vi "test_5772_stage2.vi"() -> ()   [LabVIEW 2013]
uses:
  <vilib>/measure/maspectr.llb/Power Spectrum and PSD Export Mode.ctl
  <vilib>/measure/maspectr.llb/FFT Power Spectrum and PSD for 1 Chan (CDB).vi
  <vilib>/measure/NI_MAPro.lvlib
  <vilib>/rvi/FXPMathLib/FxpInterpret/XNode/nifxpmath_Interpret.xnode
panel:
  out "size before":i32
  out "data in":dbl[](graph)
  out "size after":i32
  out "power spectrum after":cluster{"f0":dbl, "df":dbl, "magnitude":dbl[]}(graph)
  out "power spectrum bef":cluster{"f0":dbl, "df":dbl, "magnitude":dbl[]}(graph)
  out "data out":i16[](graph)
  out "Iteration":i32
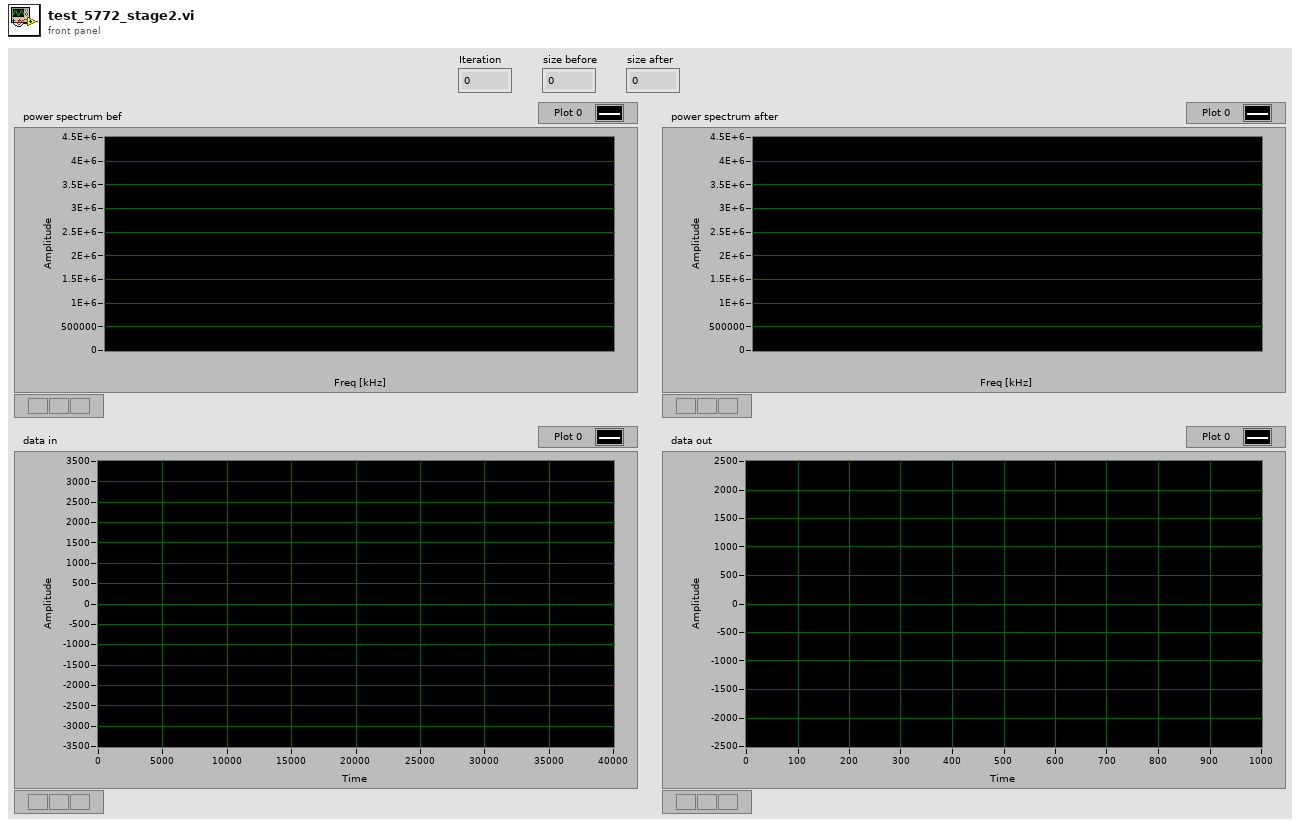
[diagram p1: front panel]
types:
  T1 = typedef "NI_MAPro.lvlib/Power Spectrum and PSD Export Mode.ctl" = u16
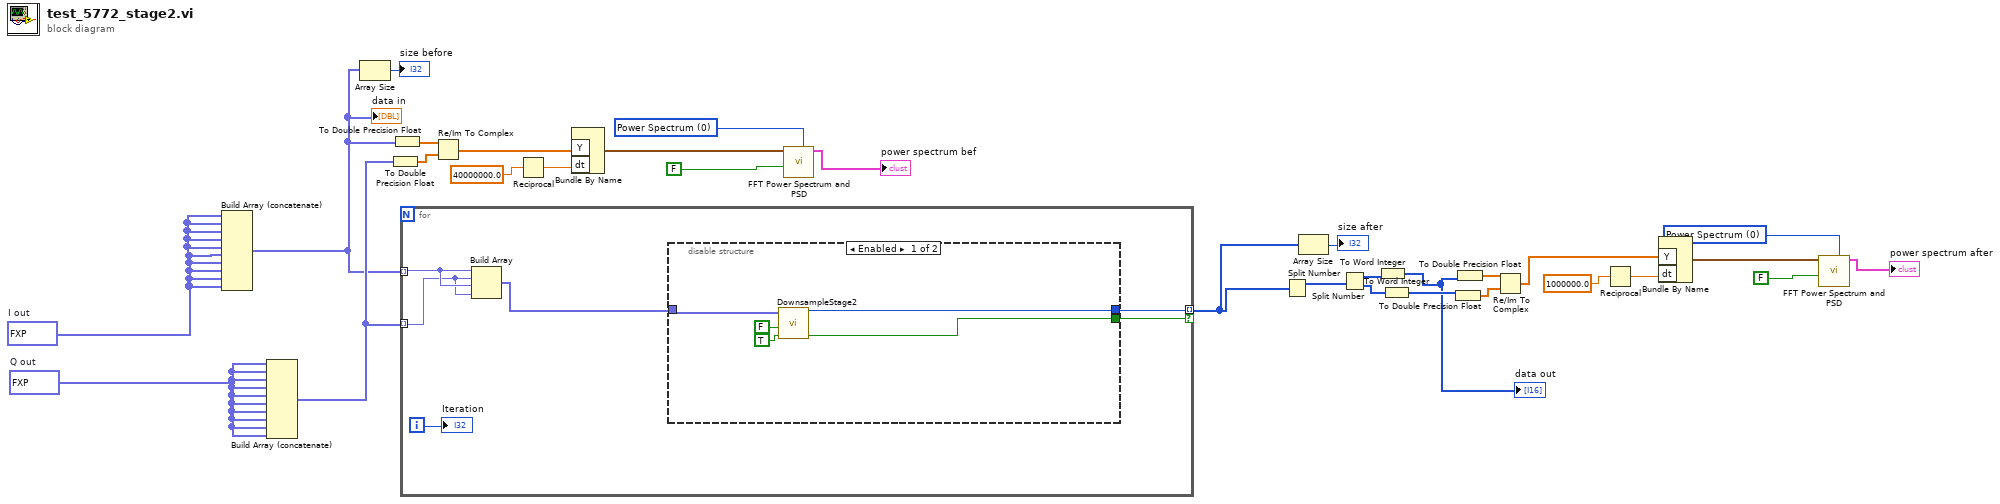
[diagram p0: block diagram]
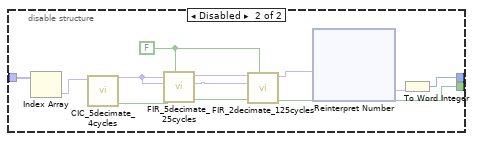
[diagram p2: hidden frame]
diagram:
  w4 = fxp[] data[31948B]  # Q out
  w5 = fxp[] data[31948B]  # I out
  w16 = T1 0 items=["Power Spectrum", "Power Spectral Density"] ("export mode")
  w30 = T1 0 items=["Power Spectrum", "Power Spectral Density"] ("export mode")
  n1 = Build Array (concatenate)(w5, w5, w5, w5, w5, w5, w5, w5, w5, w5) -> (w1:fxp<+/-,16,14>[])
  "data in" <- w1
  n2 = Build Array (concatenate)(w4, w4, w4, w4, w4, w4, w4, w4, w4, w4) -> (w6:fxp<+/-,16,14>[])
  n3 = Array Size(array=w1) -> (size(s)=→"size before":i32)
  n4 = To Double Precision Float(number=w6) -> (double precision float=w23:dbl[])
  n5 = To Double Precision Float(number=w1) -> (double precision float=w24:dbl[])
  n6 = for {
    tunnel: w1 -> [w36] mode=indexing
    tunnel: w6 -> [w35] mode=indexing
    tunnel: [w32] -> w3 mode=indexing if=w31
    i -> [w34]
    n7 = Build Array(w36, w35, w36, w35) -> (w33:fxp<+/-,16,14>[])
    n8 = disable-structure shown="Enabled" {
      disable-tunnel: w33 -> [w39 w48]
      disable-tunnel: [w40 w46] -> w31
      disable-tunnel: [w37 w43] -> w32
      frame Enabled {
        n9 = call "DownsampleStage2.vi"("valid in"=TRUE, "reset"=FALSE, "Element"=w39) -> ("valid out"=w40:bool, "Element"=w37:u64)  [unwired: 7 in]
      }
      frame Disabled {
        w50 = FALSE ("reset")
        n10 = Index Array(array=w48) -> (element=w47:fxp<+/-,16,14>)  [unwired: 1 in]
        n11 = call "CIC_5decimate_4cycles.vi"("Data in"=w47) -> ("valid out"=w53:bool, "Data out"=w54:fxp<+/-,16,14>, "valid in"=w42:bool)  [unwired: 7 in, 1 out]
        n12 = call "FIR_5decimate_25cycles.vi"("reset"=w50, "valid in"=w53, "Q in"=w54, "I in"=w54) -> ("valid out"=w49:bool, "Q out"=w51:fxp<+/-,16,14>, "I out"=w52:fxp<+/-,16,14>)  [unwired: 4 in, 1 out]
        n13 = call "FIR_2decimate_125cycles.vi"("reset"=w50, "valid in"=w49, "Q in"=w51, "I in"=w52) -> ("valid out"=w46:bool, "I out"=w44:fxp<+/-,16,14>)  [unwired: 4 in, 2 out]
        n14 = xnode "Reinterpret Number"("x"=w44) -> ("y"=w45:fxp<+/-,16,16>)
        n15 = To Word Integer(number=w45) -> (16bit integer=w43:i16)
      }
    }
    "Iteration" <- w34
  }
  n16 = Re/Im To Complex(1:w23, 2:w24) -> (0:w22:cdb[])
  n17 = Reciprocal(x=40000000.0 ("dt")) -> (1/x=w26:dbl)
  n18 = Bundle By Name("Y"=w22, "dt"=w26) -> (w29:waveform(cdb))  [unwired: 1 in]
  n19 = call-poly <vilib>:"FFT Power Spectrum and PSD.vi"("export mode"=w30, "dB On (F)"=FALSE, "time signal"=w29) -> ("Power Spectrum / PSD"=→"power spectrum bef":cluster{"f0":dbl, "df":dbl, "magnitude":dbl[]})  [unwired: 5 in, 3 out]
  n20 = Split Number(x=w3) -> (hi(x)=w12:u32[])  [unwired: 1 out]
  n21 = Array Size(array=w3) -> (size(s)=→"size after":i32)
  n22 = Split Number(x=w12) -> (hi(x)=w11:u16[], lo(x)=w10:u16[])
  n23 = To Word Integer(number=w11) -> (16bit integer=w8:i16[])
  "data out" <- w8
  n24 = To Word Integer(number=w10) -> (16bit integer=w9:i16[])
  n25 = To Double Precision Float(number=w9) -> (double precision float=w15:dbl[])
  n26 = To Double Precision Float(number=w8) -> (double precision float=w14:dbl[])
  n27 = Re/Im To Complex(1:w15, 2:w14) -> (0:w13:cdb[])
  n28 = Reciprocal(x=1000000.0 ("dt")) -> (1/x=w20:dbl)
  n29 = Bundle By Name("Y"=w13, "dt"=w20) -> (w17:waveform(cdb))  [unwired: 1 in]
  n30 = call-poly <vilib>:"FFT Power Spectrum and PSD.vi"("export mode"=w16, "dB On (F)"=FALSE, "time signal"=w17) -> ("Power Spectrum / PSD"=→"power spectrum after":cluster{"f0":dbl, "df":dbl, "magnitude":dbl[]})  [unwired: 5 in, 3 out]
